vi "De-embed S-parameters.vi"() -> ()   [LabVIEW 2020]
panel:
  out "error out":errorcluster
  in  "In Use Left":bool caption="In Use"
  in  "Swap Ports Left":bool caption="Swap Ports"
  in  "System OK Button":bool
  in  "System Stop Button":bool
  in  "In Use Right":bool caption="In Use"
  in  "De-embed":bool=TRUE
  in  "Truncate files":bool
  in  "Truncate index":i32
  in  "Ignore lowest frequency point (ISD discards it)":bool
  in  "Swap Ports Right":bool caption="Swap Ports"
  out "Horizontal Progress Bar":u8(slide) scale=0.0..100.0
  in  "Use left file":bool
  in  "(De-)embedding file right":path
  in  "(De-)embedding file left":path
  in  "DUT+Fixture":path caption="DUT+Fixture (folder or s2p-file)"
  # "1"
  # "2"
  # "1"
  # "2"
  # "2"
  # "1"
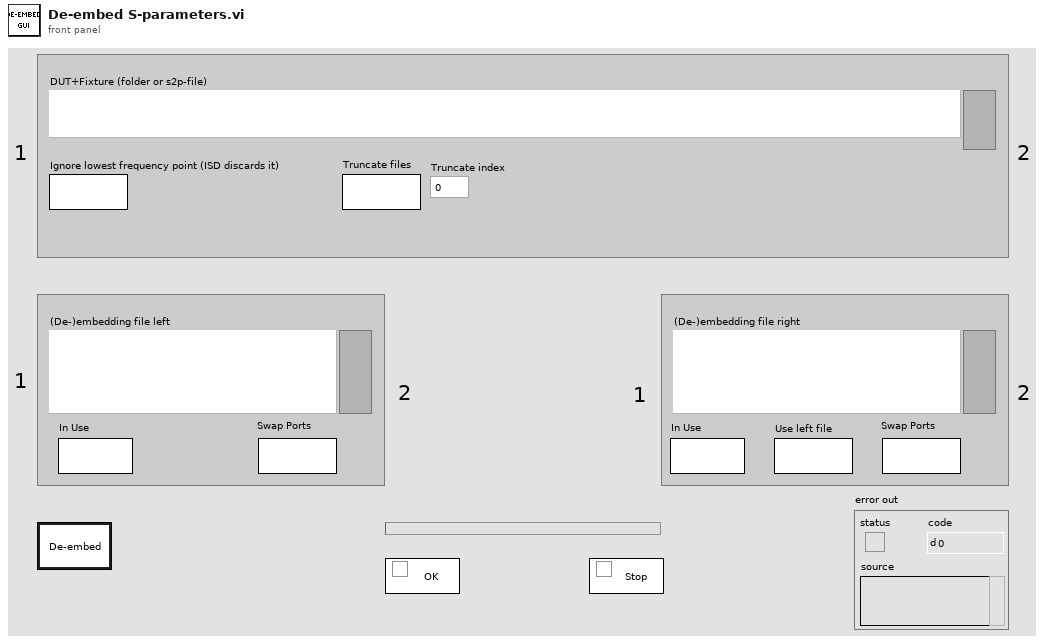
[diagram p1: front panel]
types:
  T1 = cluster{"(De-)embedding file":path, "S-parameters":cdb[][], "Frequencies (Hz)":dbl[], "output string":string, "Use":bool, "Swap Ports":bool, "De-embed":bool}
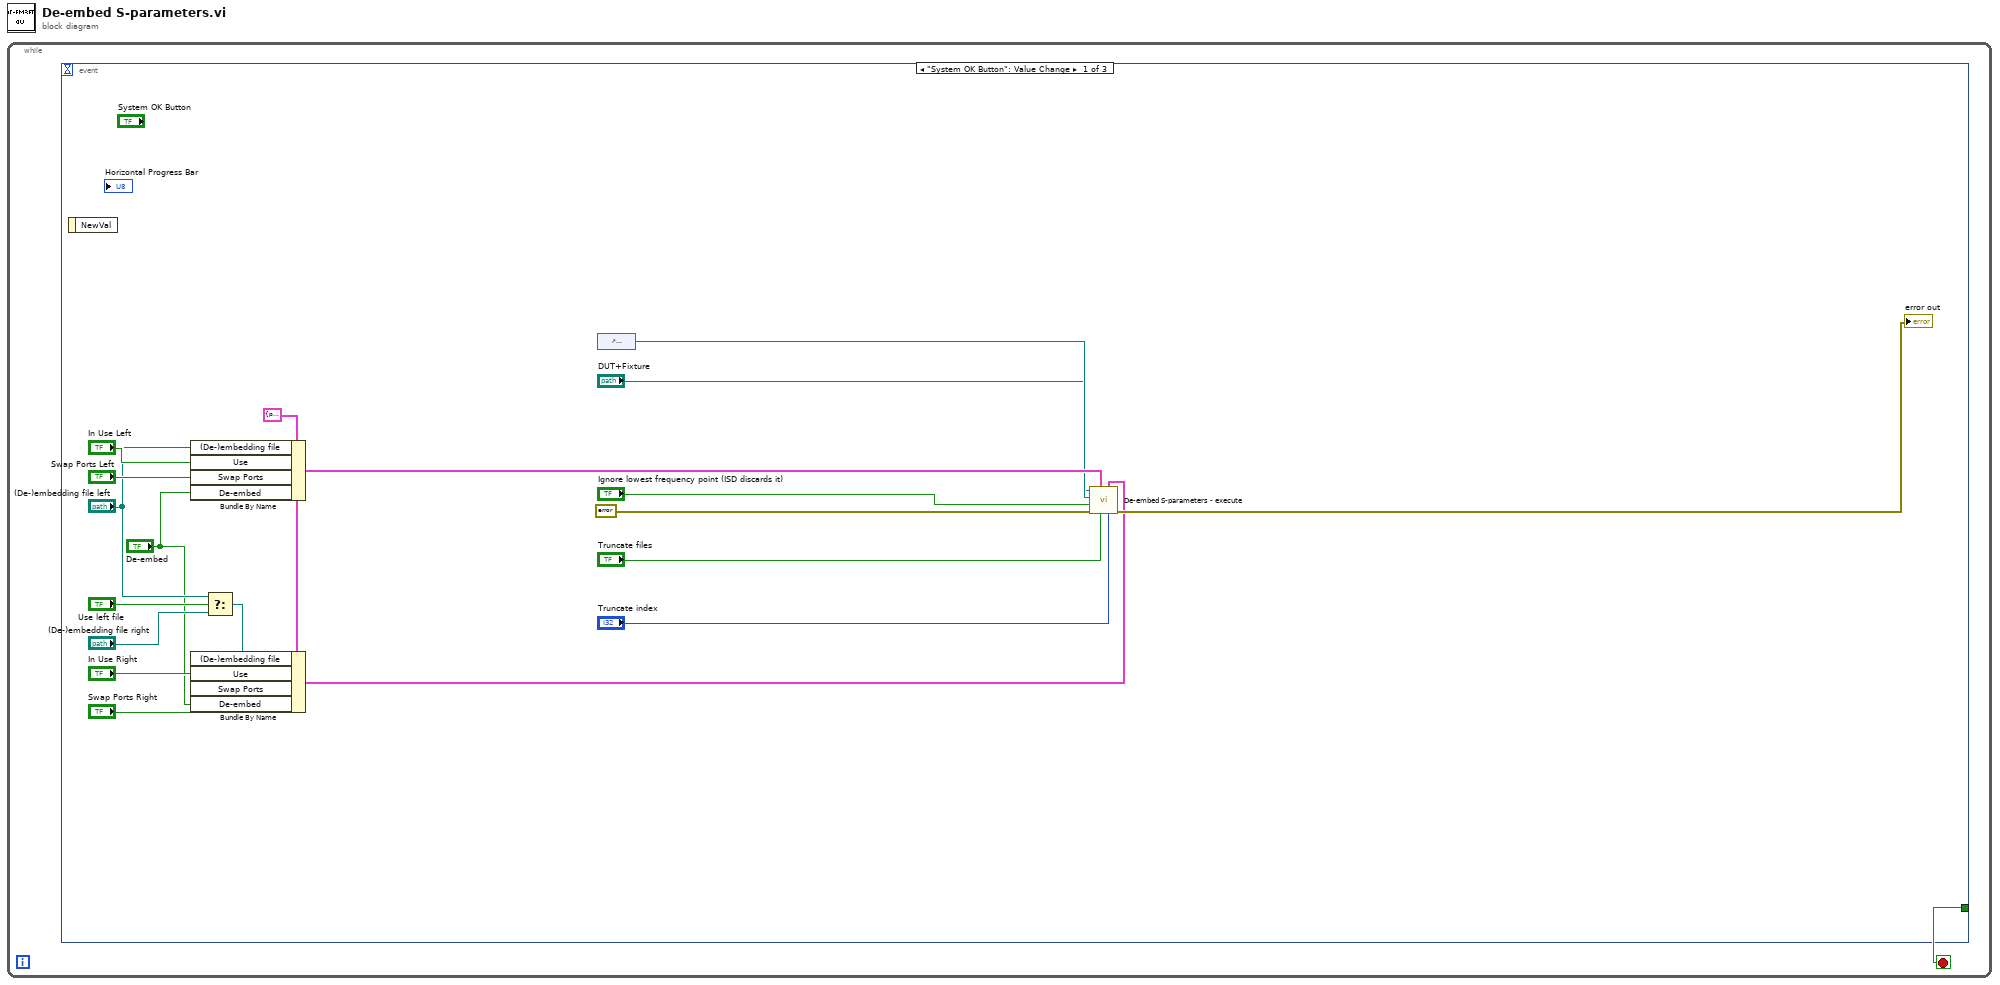
[diagram p0: block diagram]
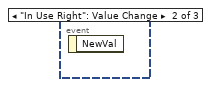
[diagram p2: hidden frame]
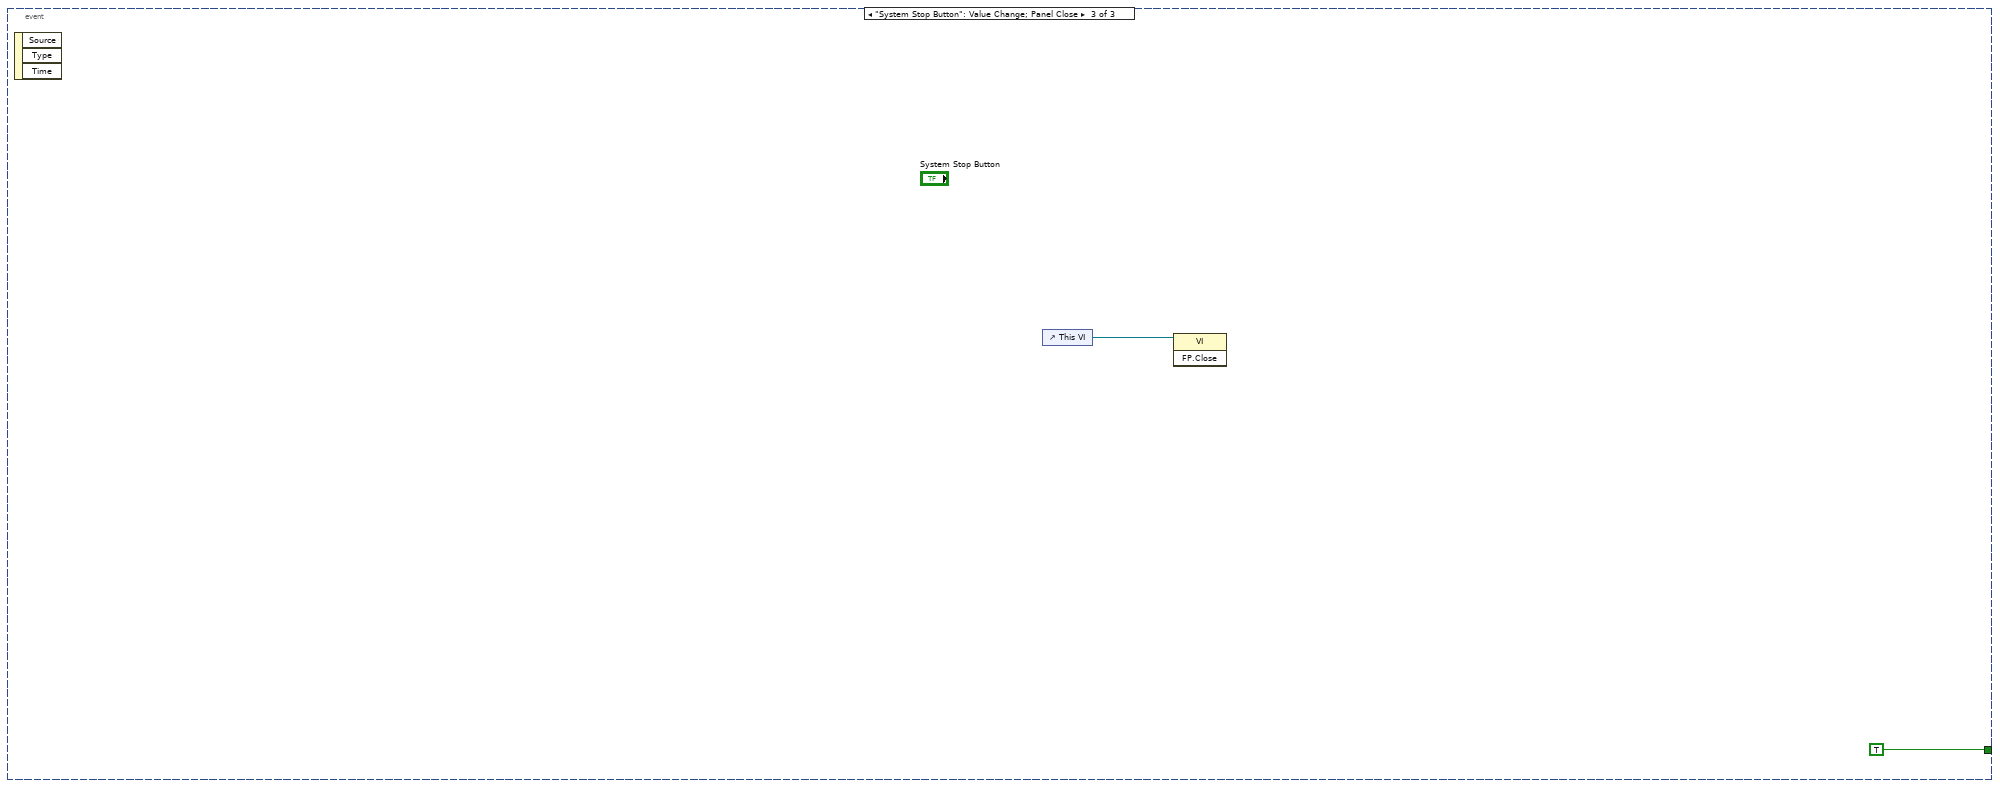
[diagram p3: hidden frame]
diagram:
  n1 = while {
    stop <- w1 stop-if-true
    n2 = event shown="[0] \"System OK Button\": Value Change" {
      selector: _ -> [_ _ _]
      dyn-events: _ -> [_ _ _]
      timeout: _ -> [_ _ _]
      tunnel: [_ _ TRUE] -> w1
      event "System OK Button": Value Change {
        w19 = T1 {"(De-)embedding file"=path "", "S-parameters"=[], "Frequencies (Hz)"=[], "output string"="", "Use"=TRUE, "Swap Ports"=FALSE, "De-embed"=TRUE} ("output cluster")
        n3 = event-data() -> ()  [unwired: 1 in, 1 out]
        n4 = Bundle By Name(cluster=w19, "(De-)embedding file"="(De-)embedding file left", "Use"="In Use Left", "Swap Ports"="Swap Ports Left", "De-embed"="De-embed") -> (w8:T1)
        n5 = Select(t="(De-)embedding file left", s="Use left file", f="(De-)embedding file right") -> (s? t:f=w15:path)
        n6 = Bundle By Name(cluster=w19, "(De-)embedding file"=w15, "Use"="In Use Right", "Swap Ports"="Swap Ports Right", "De-embed"="De-embed") -> (w7:T1)
        n7 = control-ref of="Horizontal Progress Bar"() -> (w3:refnum<vi>)
        n8 = call "De-embed S-parameters - execute.vi"("Truncate index"="Truncate index", "Right info"=w7, "Truncate files"="Truncate files", "Left info"=w8, "error in (no error)"=errorcluster {"status"=FALSE, "code"=0, "source"=""} ("error IO"), "Ignore lowest freq"="Ignore lowest frequency point (ISD discards it)", "Horizontal Progress Bar"=w3, "DUT+Fixture"="DUT+Fixture") -> ("error out"=→"error out":errorcluster)  [unwired: 3 in]
      }
      event "In Use Right": Value Change {
        n9 = event-data() -> ()  [unwired: 1 in, 1 out]
      }
      event "System Stop Button": Value Change; Panel Close {
        n10 = event-data() -> ()  [unwired: 1 in, 3 out]
        n11 = control-ref of="This VI"() -> (w21:refnum<vi>)
        n12 = invoke class="VI" method="FP.Close"(reference=w21) -> ()  [unwired: 2 in, 3 out]
      }
    }
  }
